vi "Test shm register Callback command wait ackcmd LV.vi"(8 "error in (no error)":errorcluster, 10 "skipOld":bool, 11 "handle":i32) -> (0 "error out":errorcluster, 3 "function return":i32)   [LabVIEW 2018, in "SALLV_Test.lvlib"]
doc: "int Test_shm_registerCallback_command_wait_ackcmdLV(int handle, bool skipOld);"
uses:
  SALLV_Test.lvlib
  SALLV_Test.so
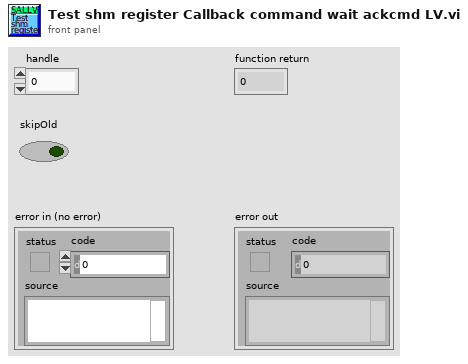
[diagram p1: front panel]
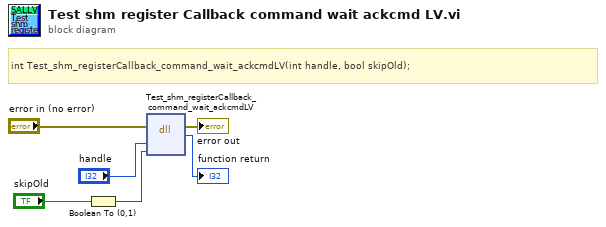
[diagram p0: block diagram]
diagram:
  # "int Test_shm_registerCallback_command_wait_ackcmdLV(int handle, bool skipOld);"
  n1 = Boolean To (0,1)(Boolean="skipOld") -> (0, 1=w3:i16)
  n2 = dll-call lib="home/ttsai/Documents/salLabVIEWtestData/SALLV_Test.*" fn="Test_shm_registerCallback_command_wait_ackcmdLV"(error in="error in (no error)", "handle"="handle", "skipOld"=w3) -> (error out=→"error out":errorcluster, →"function return":i32)  [unwired: 4 in, 1 out]
